vi "Node_ID_AlarmCMD.vi"(5 "error in":errorcluster) -> (10 "Node ID":string[](array[string]), 11 "appended array":string[](array[string]), 12 "TotalMain1":string[](array[string]), 13 "TotalMain2":string[](array[string]), 14 "Main 1":string[](array[string]), 15 "Main 2":string[](array[string]), 16 "Fork Node":string[](array[string]), 17 "Tube":string[](array[string]), 18 "UT":string[](array[string]), 19 "error out":errorcluster)   [LabVIEW 2019]
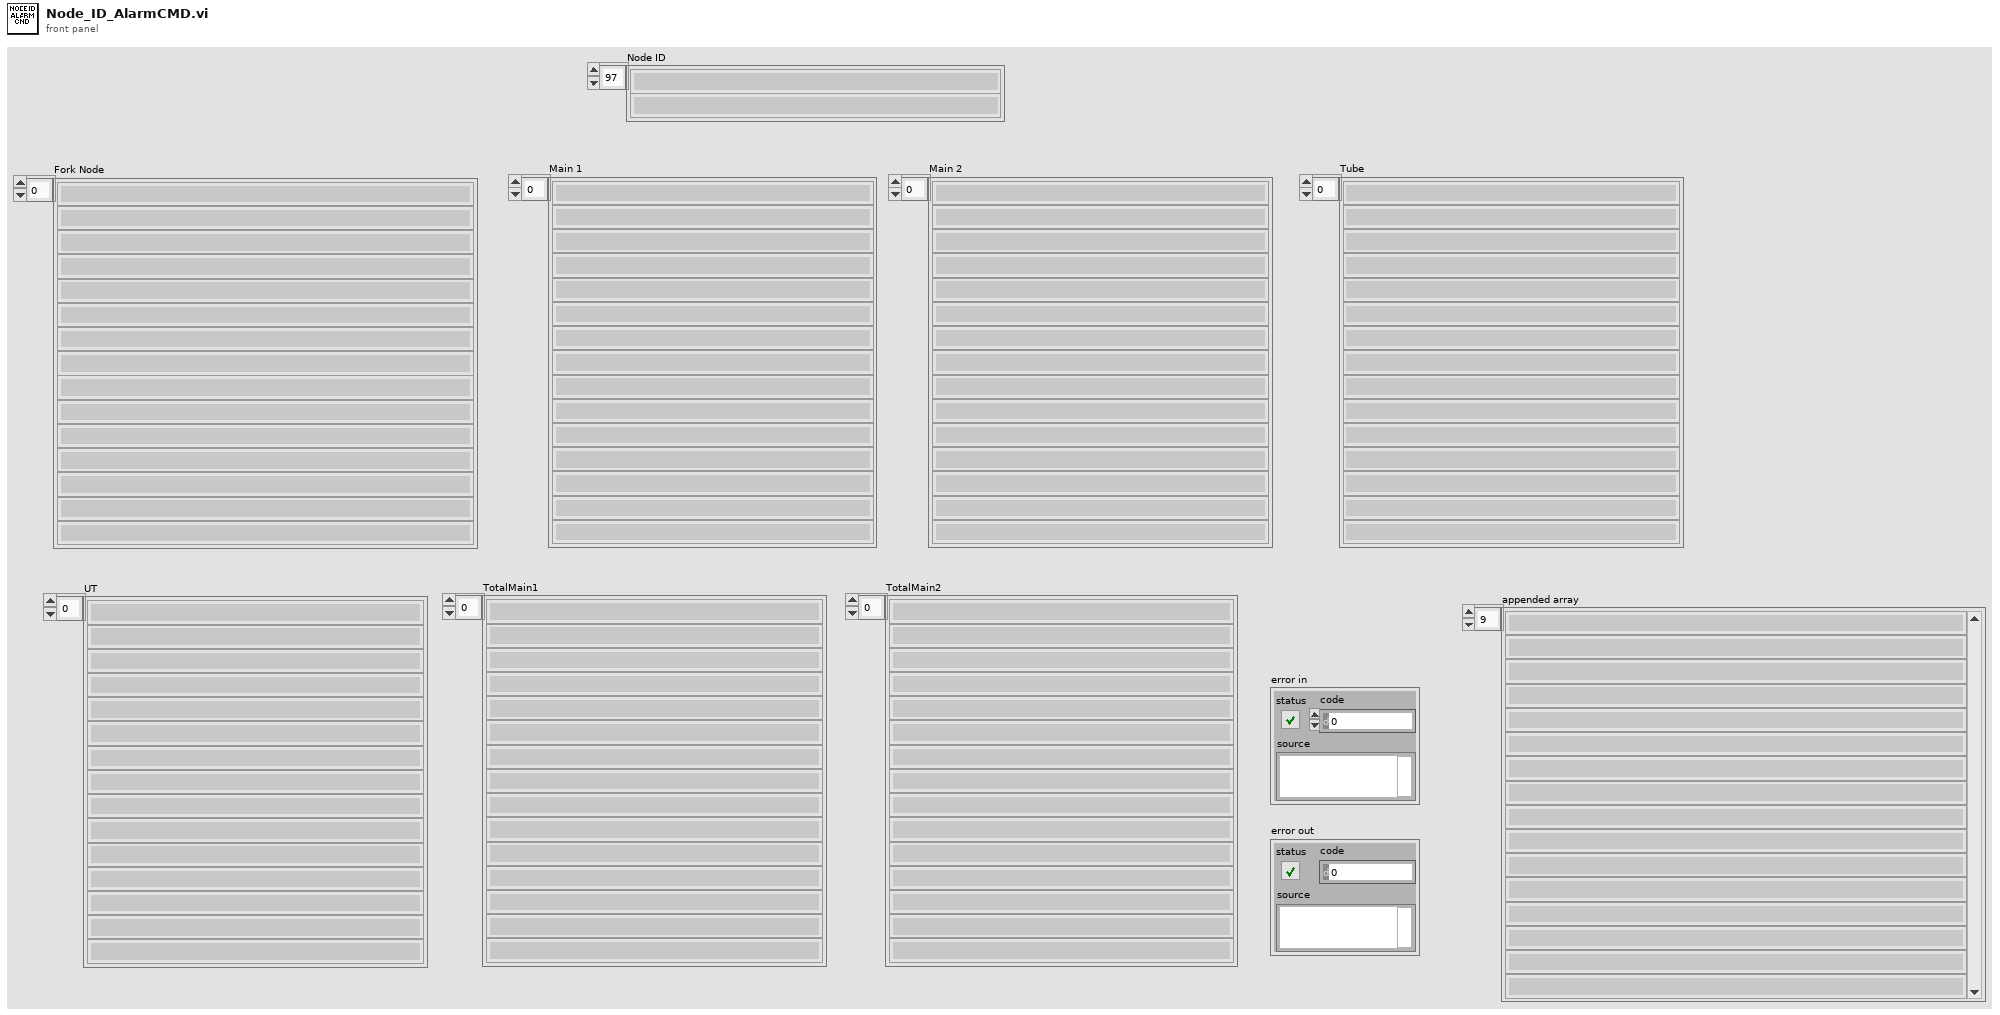
[diagram p1: front panel]
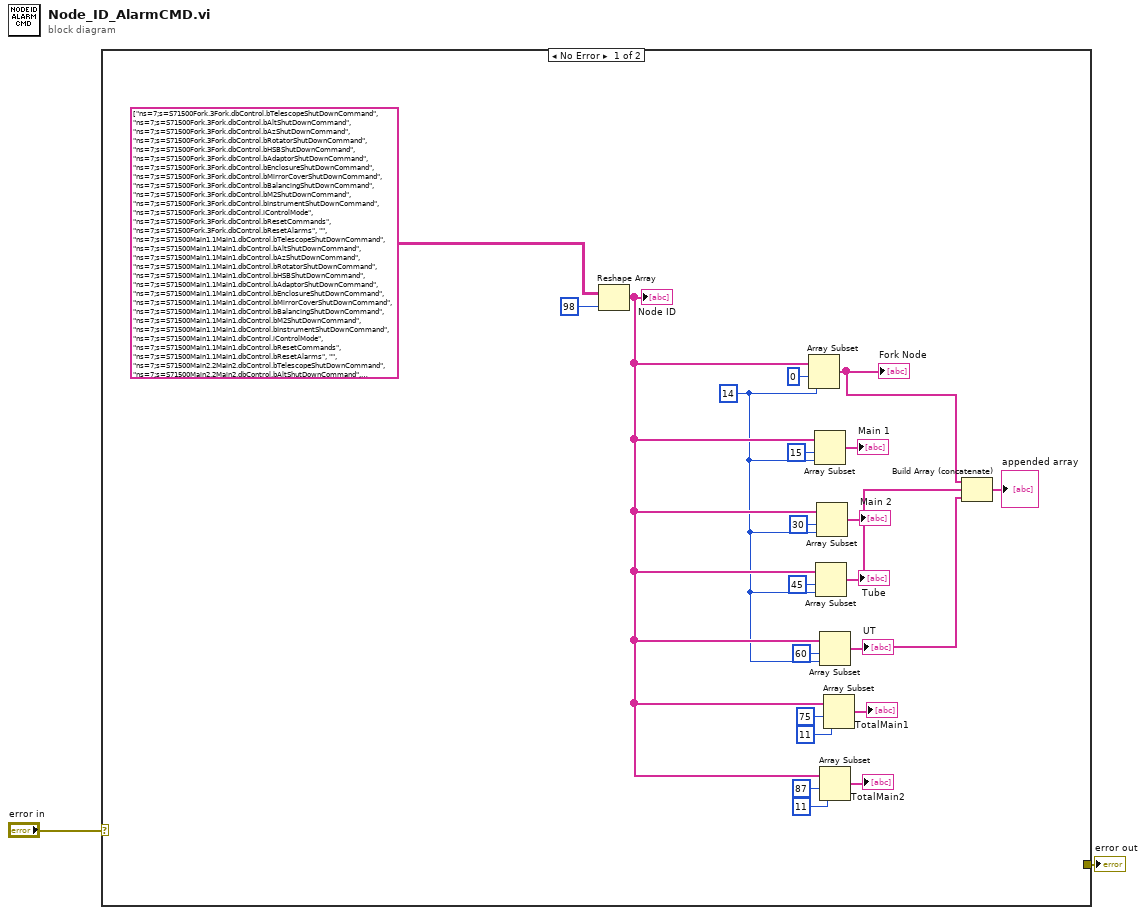
[diagram p0: block diagram]
diagram:
  n1 = case shown="No Error" "error in" {
    selector: "error in" -> [_ w24]
    tunnel: [_ w24] -> w1
    frame No Error {
      w9 = 14 ("length")
      n2 = Reshape Array(string[][] [["ns=7;s=S71500Fork.3Fork.dbControl.bTelescopeShutDownCommand"], ["ns=7;s=S71500Fork.3Fork.dbControl.bAltShutDownCommand"], ["ns=7;s=S71500Fork.3Fork.dbControl.bAzShutDownCommand"], ["ns=7;s=S71500Fork.3Fork.dbControl.bRotatorShutDownCommand"], ["ns=7;s=S71500Fork.3Fork.dbControl.bHSBShutDownCommand"], ["ns=7;s=S71500Fork.3Fork.dbControl.bAdaptorShutDownCommand"], ["ns=7;s=S71500Fork.3Fork.dbControl.bEnclosureShutDownCommand"], ["ns=7;s=S71500Fork.3Fork.dbControl.bMirrorCoverShutDownCommand"], ["ns=7;s=S71500Fork.3Fork.dbControl.bBalancingShutDownCommand"], ["ns=7;s=S71500Fork.3Fork.dbControl.bM2ShutDownCommand"], ["ns=7;s=S71500Fork.3Fork.dbControl.bInstrumentShutDownCommand"], ["ns=7;s=S71500Fork.3Fork.dbControl.iControlMode"], ["ns=7;s=S71500Fork.3Fork.dbControl.bResetCommands"], ["ns=7;s=S71500Fork.3Fork.dbControl.bResetAlarms"], [""], ["ns=7;s=S71500Main1.1Main1.dbControl.bTelescopeShutDownCommand"], ["ns=7;s=S71500Main1.1Main1.dbControl.bAltShutDownCommand"], ["ns=7;s=S71500Main1.1Main1.dbControl.bAzShutDownCommand"], ["ns=7;s=S71500Main1.1Main1.dbControl.bRotatorShutDownCommand"], ["ns=7;s=S71500Main1.1Main1.dbControl.bHSBShutDownCommand"], ["ns=7;s=S71500Main1.1Main1.dbControl.bAdaptorShutDownCommand"], ["ns=7;s=S71500Main1.1Main1.dbControl.bEnclosureShutDownCommand"], ["ns=7;s=S71500Main1.1Main1.dbControl.bMirrorCoverShutDownCommand"], ["ns=7;s=S71500Main1.1Main1.dbControl.bBalancingShutDownCommand"], ["ns=7;s=S71500Main1.1Main1.dbControl.bM2ShutDownCommand"], ["ns=7;s=S71500Main1.1Main1.dbControl.bInstrumentShutDownCommand"], ["ns=7;s=S71500Main1.1Main1.dbControl.iControlMode"], ["ns=7;s=S71500Main1.1Main1.dbControl.bResetCommands"], ["ns=7;s=S71500Main1.1Main1.dbControl.bResetAlarms"], [""], ["ns=7;s=S71500Main2.2Main2.dbControl.bTelescopeShutDownCommand"], ["ns=7;s=S71500Main2.2Main2.dbControl.bAltShutDownCommand"], ["ns=7;s=S71500Main2.2Main2.dbControl.bAzShutDownCommand"], ["ns=7;s=S71500Main2.2Main2.dbControl.bRotatorShutDownCommand"], ["ns=7;s=S71500Main2.2Main2.dbControl.bHSBShutDownCommand"], ["ns=7;s=S71500Main2.2Main2.dbControl.bAdaptorShutDownCommand"], ["ns=7;s=S71500Main2.2Main2.dbControl.bEnclosureShutDownCommand"], ["ns=7;s=S71500Main2.2Main2.dbControl.bMirrorCoverShutDownCommand"], ["ns=7;s=S71500Main2.2Main2.dbControl.bBalancingShutDownCommand"], ["ns=7;s=S71500Main2.2Main2.dbControl.bM2ShutDownCommand"], ["ns=7;s=S71500Main2.2Main2.dbControl.bInstrumentShutDownCommand"], ["ns=7;s=S71500Main2.2Main2.dbControl.iControlMode"], ["ns=7;s=S71500Main2.2Main2.dbControl.bResetCommands"], ["ns=7;s=S71500Main2.2Main2.dbControl.bResetAlarms"], [""], ["ns=7;s=S71500Tube.4Tube.dbControl.bTelescopeShutDownCommand"], ["ns=7;s=S71500Tube.4Tube.dbControl.bAltShutDownCommand"], ["ns=7;s=S71500Tube.4Tube.dbControl.bAzShutDownCommand"], ["ns=7;s=S71500Tube.4Tube.dbControl.bRotatorShutDownCommand"], ["ns=7;s=S71500Tube.4Tube.dbControl.bHSBShutDownCommand"], ["ns=7;s=S71500Tube.4Tube.dbControl.bAdaptorShutDownCommand"], ["ns=7;s=S71500Tube.4Tube.dbControl.bEnclosureShutDownCommand"], ["ns=7;s=S71500Tube.4Tube.dbControl.bMirrorCoverShutDownCommand"], ["ns=7;s=S71500Tube.4Tube.dbControl.bBalancingShutDownCommand"], ["ns=7;s=S71500Tube.4Tube.dbControl.bM2ShutDownCommand"], ["ns=7;s=S71500Tube.4Tube.dbControl.bInstrumentShutDownCommand"], ["ns=7;s=S71500Tube.4Tube.dbControl.iControlMode"], ["ns=7;s=S71500Tube.4Tube.dbControl.bResetCommands"], ["ns=7;s=S71500Tube.4Tube.dbControl.bResetAlarms"], [""], ["ns=7;s=S71500UT.5UT.dbControl.bTelescopeShutDownCommand"], ["ns=7;s=S71500UT.5UT.dbControl.bAltShutDownCommand"], ["ns=7;s=S71500UT.5UT.dbControl.bAzShutDownCommand"], ["ns=7;s=S71500UT.5UT.dbControl.bRotatorShutDownCommand"], ["ns=7;s=S71500UT.5UT.dbControl.bHSBShutDownCommand"], ["ns=7;s=S71500UT.5UT.dbControl.bAdaptorShutDownCommand"], ["ns=7;s=S71500UT.5UT.dbControl.bEnclosureShutDownCommand"], ["ns=7;s=S71500UT.5UT.dbControl.bMirrorCoverShutDownCommand"], ["ns=7;s=S71500UT.5UT.dbControl.bBalancingShutDownCommand"], ["ns=7;s=S71500UT.5UT.dbControl.bM2ShutDownCommand"], ["ns=7;s=S71500UT.5UT.dbControl.bInstrumentShutDownCommand"], ["ns=7;s=S71500UT.5UT.dbControl.iControlMode"], ["ns=7;s=S71500UT.5UT.dbControl.bResetCommands"], ["ns=7;s=S71500UT.5UT.dbControl.bResetAlarms"], [""], ["ns=7;s=S71500Main1.1Main1.dbTotalCommand.bTelescopeShutDownCommand"], ["ns=7;s=S71500Main1.1Main1.dbTotalCommand.bAltShutDownCommand"], ["ns=7;s=S71500Main1.1Main1.dbTotalCommand.bAzShutDownCommand"], ["ns=7;s=S71500Main1.1Main1.dbTotalCommand.bRotatorShutDownCommand"], ["ns=7;s=S71500Main1.1Main1.dbTotalCommand.bHSBShutDownCommand"], ["ns=7;s=S71500Main1.1Main1.dbTotalCommand.bAdaptorShutDownCommand"], ["ns=7;s=S71500Main1.1Main1.dbTotalCommand.bEnclosureShutDownCommand"], ["ns=7;s=S71500Main1.1Main1.dbTotalCommand.bMirrorCoverShutDownCommand"], ["ns=7;s=S71500Main1.1Main1.dbTotalCommand.bBalancingShutDownCommand"], ["ns=7;s=S71500Main1.1Main1.dbTotalCommand.bM2ShutDownCommand"], ["ns=7;s=S71500Main1.1Main1.dbTotalCommand.bInstrumentShutDownCommand"], [""], ["ns=7;s=S71500Main2.2Main2.dbTotalCommand.bResetCommands"], ["ns=7;s=S71500Main2.2Main2.dbTotalCommand.bResetAlarms"], ["ns=7;s=S71500Main2.2Main2.dbTotalCommand.bTelescopeShutDownCommand"], ["ns=7;s=S71500Main2.2Main2.dbTotalCommand.bAltShutDownCommand"], ["ns=7;s=S71500Main2.2Main2.dbTotalCommand.bAzShutDownCommand"], ["ns=7;s=S71500Main2.2Main2.dbTotalCommand.bRotatorShutDownCommand"], ["ns=7;s=S71500Main2.2Main2.dbTotalCommand.bHSBShutDownCommand"], ["ns=7;s=S71500Main2.2Main2.dbTotalCommand.bAdaptorShutDownCommand"], ["ns=7;s=S71500Main2.2Main2.dbTotalCommand.bEnclosureShutDownCommand"], ["ns=7;s=S71500Main2.2Main2.dbTotalCommand.bMirrorCoverShutDownCommand"], ["ns=7;s=S71500Main2.2Main2.dbTotalCommand.bBalancingShutDownCommand"], [""]] ("data"), 98 ("dimension size")) -> (w10:string[])
      "Node ID" <- w10
      n3 = Array Subset(array=w10, index=0, length=w9) -> (w4:string[])
      "Fork Node" <- w4
      n4 = Array Subset(array=w10, index=15, length=w9) -> (→"Main 1":string[])
      n5 = Array Subset(array=w10, index=45, length=w9) -> (w6:string[])
      "Tube" <- w6
      n6 = Array Subset(array=w10, index=30, length=w9) -> (→"Main 2":string[])
      n7 = Array Subset(array=w10, index=60, length=w9) -> (w5:string[])
      "UT" <- w5
      n8 = Array Subset(array=w10, index=87, length=11) -> (→"TotalMain2":string[])
      n9 = Array Subset(array=w10, index=75, length=11) -> (→"TotalMain1":string[])
      n10 = Build Array (concatenate)(w4, w6, w5) -> (→"appended array":string[])
    }
    frame Error {
    }
  }
  "error out" <- w1
